vi "Get Attribute Name and Parent ID.vi"(8 "error in (no error)":errorcluster, 10 "Tag":string, 11 "Test Executive in":refnum<class "Test Executive.lvclass">) -> (0 "error out":errorcluster, 1 "Attribute Name":string, 2 "Parent ID":string, 3 "Test Executive out":refnum<class "Test Executive.lvclass">)   [LabVIEW 2017, in "Test Executive.lvlib" / "Test Executive.lvclass"]
uses:
  <vilib>/gpm_packages/@cs/test-executive/Source/Test Executive/TestExecutive/Test Executive.lvclass
  <vilib>/gpm_packages/@cs/test-executive/Source/Test Executive/TestExecutive/Test Executive.lvclass/Test Executive.ctl
  <vilib>/gpm_packages/@cs/linked-list/Source/Linked List/Linked List Ref/Linked List Ref.lvclass
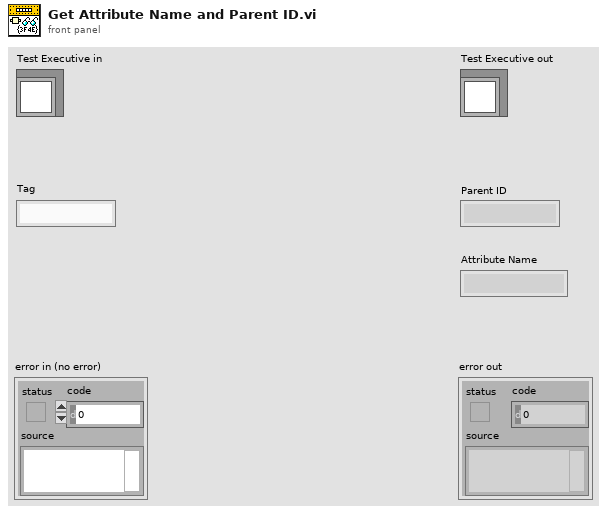
[diagram p1: front panel]
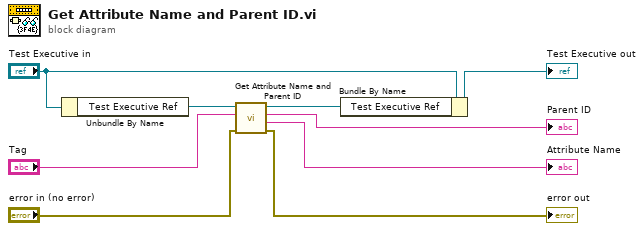
[diagram p0: block diagram]
diagram:
  n1 = Unbundle By Name("Test Executive in") -> ("Test Executive Ref"=w7:refnum<data-value>)
  n2 = call <vilib>:"Get Attribute Name and Parent ID.vi"("error in (no error)"="error in (no error)", "Tag"="Tag", "Linked List Ref"=w7) -> ("error out"=→"error out":errorcluster, "Attribute Name"=→"Attribute Name":string, "Linked List ID"=→"Parent ID":string, "Linked List Ref out"=w6:refnum<data-value>)  [unwired: 5 in]
  n3 = Bundle By Name(cluster="Test Executive in", "Test Executive Ref"=w6) -> (→"Test Executive out":refnum<class "Test Executive.lvclass">)
